vi "NTJ_Srv_Bld_Msg_17.vi"(10 "Field Value":T1, 11 "Field ID":T4) -> (3 "Msg Buffer":string)   [LabVIEW 2019]
uses:
  <vilib>/Rock Robotics/Network Tables/Field ID.ctl
  <vilib>/Rock Robotics/Network Tables/Field Data.ctl
  <vilib>/Rock Robotics/Network Tables/Field Type.ctl
  <vilib>/Rock Robotics/Network Tables/Sequence.ctl
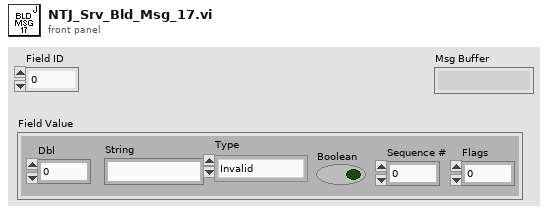
[diagram p1: front panel]
types:
  T1 = typedef "Field Data.ctl" = cluster{"Dbl":dbl, "String":string, "Type":T2, "Boolean":bool, "Sequence #":T3, "Flags":u8}
  T2 = typedef "Field Type.ctl" = enum8{"Invalid", "Bool", "Numeric", "String", "Raw", "Boolean Array", "Numeric Array", "String Array", "RPC"}
  T3 = typedef "Sequence.ctl" = u16
  T4 = typedef "Field ID.ctl" = i32
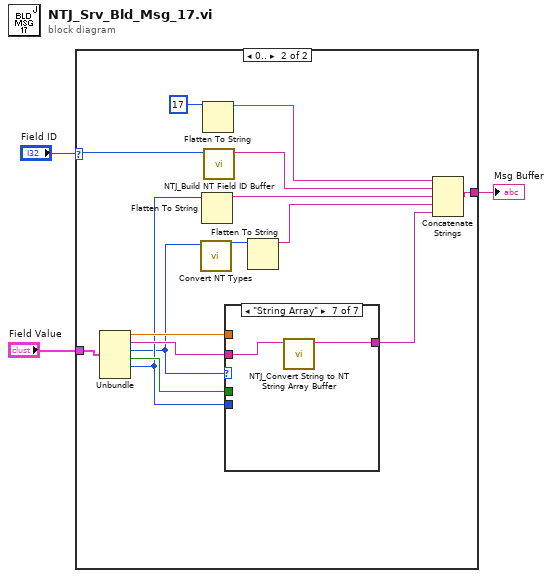
[diagram p0: block diagram]
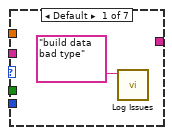
[diagram p3: hidden frame]
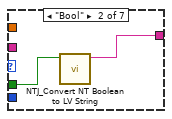
[diagram p4: hidden frame]
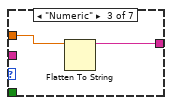
[diagram p5: hidden frame]
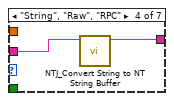
[diagram p6: hidden frame]
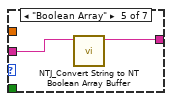
[diagram p7: hidden frame]
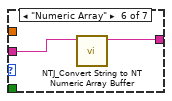
[diagram p8: hidden frame]
diagram:
  n1 = case shown="0.." "Field ID" {
    selector: "Field ID" -> [_ w8]
    tunnel: "Field Value" -> [_ w16]
    tunnel: [_ w9] -> w2
    frame Default {
    }
    frame 0.. {
      n2 = Unbundle(w16) -> ("Dbl"=w18:dbl, "String"=w17:string, "Type"=w7:T2, "Boolean"=w15:bool, "Sequence #"=w10:T3)  [unwired: 1 out]
      n3 = call <vilib>:"Convert NT Types.vi"("Type in"=w7) -> ("Type out"=w6:u8)  [unwired: 10 in]
      n4 = Flatten To String(anything=w10) -> (data string=w14:string)  [unwired: 3 in, 2 out]
      n5 = Flatten To String(anything=u8 17 ("bytes to read")) -> (data string=w13:string)  [unwired: 3 in, 2 out]
      n6 = call "NTJ_Build NT Field ID Buffer.vi"("Field ID"=w8) -> ("Data Buffer"=w11:string)  [unwired: 10 in]
      n7 = case shown="\"String Array\"" w7 {
        tunnel: w10 -> [_ _ _ _ _ _ _]
        tunnel: w17 -> [_ _ _ w25 w26 w28 w30]
        tunnel: [_ w20 w22 w24 w27 w29 w31] -> w5
        tunnel: w18 -> [_ _ w23 _ _ _ _]
        tunnel: w15 -> [_ w21 _ _ _ _ _]
        frame Default {
          n8 = call <vilib>:"Log Issues.vi"("Issue"="build data bad type") -> ()  [unwired: 11 in]
        }
        frame "Bool" {
          n9 = call "NTJ_Convert NT Boolean to LV String.vi"("Boolean"=w21) -> ("string"=w20:string)  [unwired: 10 in]
        }
        frame "Numeric" {
          n10 = Flatten To String(anything=w23) -> (data string=w22:string)  [unwired: 3 in, 2 out]
        }
        frame "String", "Raw", "RPC" {
          n11 = call "NTJ_Convert String to NT String Buffer.vi"("LV Buffer"=w25) -> ("NT Buffer"=w24:string)  [unwired: 10 in]
        }
        frame "Boolean Array" {
          n12 = call "NTJ_Convert String to NT Boolean Array Buffer.vi"("LV Buffer"=w26) -> ("NT Buffer"=w27:string)  [unwired: 10 in]
        }
        frame "Numeric Array" {
          n13 = call "NTJ_Convert String to NT Numeric Array Buffer.vi"("LV Buffer"=w28) -> ("NT Buffer"=w29:string)  [unwired: 10 in]
        }
        frame "String Array" {
          n14 = call "NTJ_Convert String to NT String Array Buffer.vi"("LV Buffer"=w30) -> ("NT Buffer"=w31:string)  [unwired: 10 in]
        }
      }
      n15 = Flatten To String(anything=w6) -> (data string=w4:string)  [unwired: 3 in, 2 out]
      n16 = Concatenate Strings(w13, w11, w14, w4, w5) -> (w9:string)
    }
  }
  "Msg Buffer" <- w2
